vi "Create Folder Structure.vi"(8 "error in (no error)":errorcluster, 11 "Process Generator In":refnum<class "Process Generator.lvclass">) -> (0 "error out":errorcluster, 3 "Process Generator Out":refnum<class "Process Generator.lvclass">)   [LabVIEW 2020, in "Process Generation.lvlib" / "Process Generator.lvclass"]
uses:
  Process Generator.lvclass
  Process Generator.lvclass/Process Generator.ctl
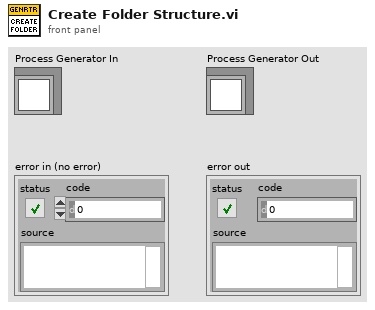
[diagram p1: front panel]
types:
  T1 = enum32{"invalid scope", "public", "private", "protected", "community"}[]
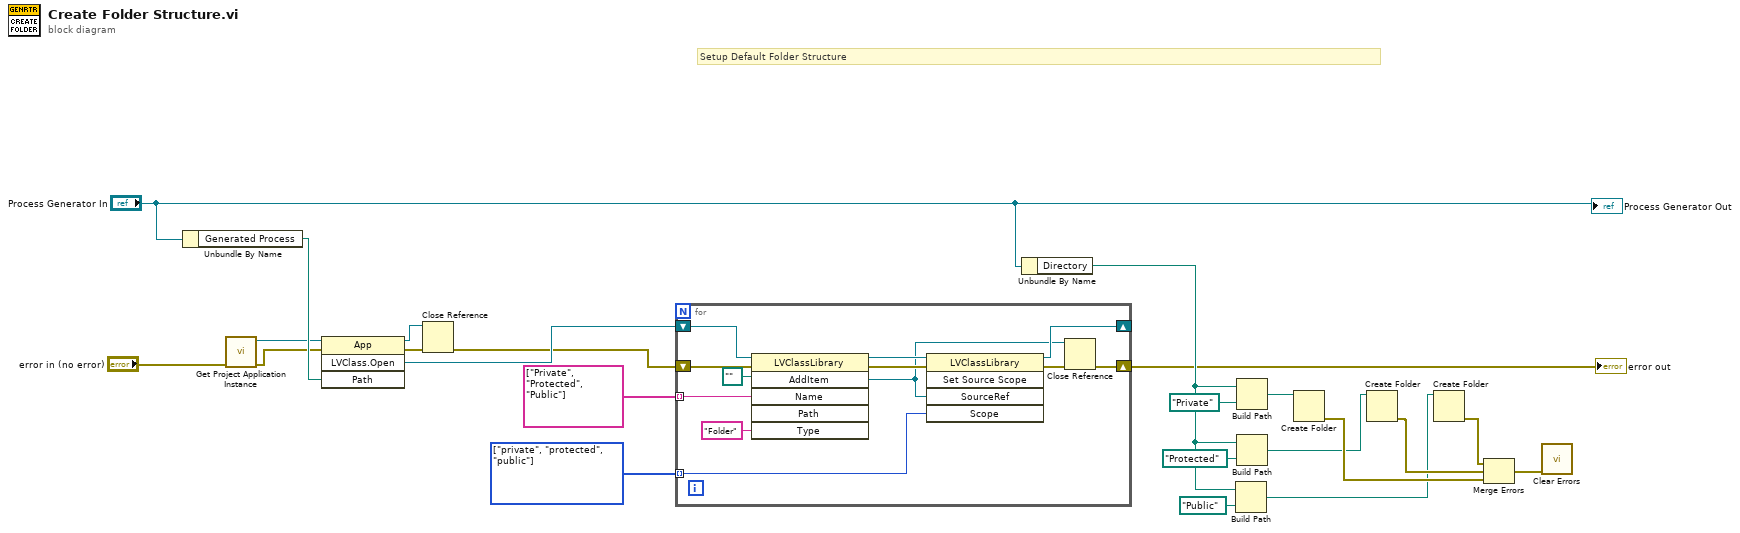
[diagram p0: block diagram]
diagram:
  w2 = T1 [enum."private", enum."protected", enum."public"] items=["invalid scope", "public", "private", "protected", "community"] ("scope")
  # "Setup Default Folder Structure"
  n1 = Unbundle By Name("Process Generator In") -> ("Generated Process"=w21:path)
  n2 = call "Get Project Application Instance.vi"("error in (no error)"="error in (no error)") -> ("error out"=w15:errorcluster, "Application out"=w14:refnum<vi>)  [unwired: 9 in]
  n3 = invoke class="App" method="LVClass.Open"(reference=w14, error in=w15, "Path"=w21) -> (reference out=w17:refnum<vi>, error out=w16:errorcluster, "LVClass.Open"=w20:refnum<vi>)  [unwired: 1 in, 1 out]
  n4 = Close Reference(reference=w17, error in (no error)=w16) -> (error out=w19:errorcluster)
  n5 = for {
    tunnel: string[] ["Private", "Protected", "Public"] ("Name") -> [w35] mode=indexing
    tunnel: w2 -> [w30] mode=indexing
    shift-right: [w29] -> _
    shift-left: w20 -> [w33]
    shift-right: [w25] -> w13
    shift-left: w19 -> [w27]
    n6 = invoke class="LVClassLibrary" method="AddItem"(reference=w33, error in=w27, "Name"=w35, "Path"=path "", "Type"="Folder") -> (reference out=w31:refnum<vi>, error out=w28:errorcluster, "AddItem"=w24:refnum<vi>)  [unwired: 1 in, 3 out]
    n7 = invoke class="LVClassLibrary" method="Set Source Scope"(reference=w31, error in=w28, "SourceRef"=w24, "Scope"=w30) -> (reference out=w29:refnum<vi>, error out=w26:errorcluster)  [unwired: 1 in, 3 out]
    n8 = Close Reference(reference=w24, error in (no error)=w26) -> (error out=w25:errorcluster)
  }
  "error out" <- w13
  n9 = Unbundle By Name("Process Generator In") -> ("Directory"=w23:path)
  n10 = Build Path(base path=w23, name or relative path=path "Public") -> (appended path=w8:path)
  n11 = Build Path(base path=w23, name or relative path=path "Private") -> (appended path=w4:path)
  n12 = Build Path(base path=w23, name or relative path=path "Protected") -> (appended path=w5:path)
  n13 = Create Folder(path (use dialog)=w4) -> (error out=w11:errorcluster)  [unwired: 2 in, 2 out]
  n14 = Create Folder(path (use dialog)=w5) -> (error out=w10:errorcluster)  [unwired: 2 in, 2 out]
  n15 = Create Folder(path (use dialog)=w8) -> (error out=w9:errorcluster)  [unwired: 2 in, 2 out]
  n16 = Merge Errors(w9, w10, w11) -> (w12:errorcluster)
  n17 = call <vilib>:"Clear Errors.vi"("error in (no error)"=w12) -> ()  [unwired: 5 in, 2 out]
  "Process Generator Out" <- "Process Generator In"
